vi "Read Multiple Digital Waveforms.vi"(8 "error in (no error)":errorcluster, 9 "Timeout (10000 ms)":u32=10000, 10 "Channels":u16[](array[ring])=[0, 1] items=["POD 1", "POD 2"], 11 "VISA resource name":refnum<visa-resource-name>) -> (0 "error out":errorcluster, 2 "Digital Waveform Graph":digitalwaveform[](graph), 3 "VISA resource name out":refnum<visa-resource-name>)   [LabVIEW 2021, in "Agilent 6000 Series.lvlib"]
doc: "Initiates an acquisition on channel that you enabled with the <B>Configure Digital Channel</B> VI. The VI waits for the acquisition to complete and returns the waveform for the Source channel you specified. If the oscilloscope did not complete the acquisition within the time period you specify with the Timeout parameter, the VI returns a time out error. A common cause for a timeout error is the acquisition was not triggered. For example, the trigger level is out of range of the waveform.\n\nCall the <B>Fetch Digital Waveform</B> VI to obtain the waveforms for each of the remaining enabled Source channels without initiating another acquisition.\n\n<B>NOTE:</B>\n\nThis VI is only supported by MSO models; running this VI with a DSO model might throw an error."
uses:
  Agilent 6000 Series.lvlib
  Low Data VIs/Fetch Digital Waveform.vi
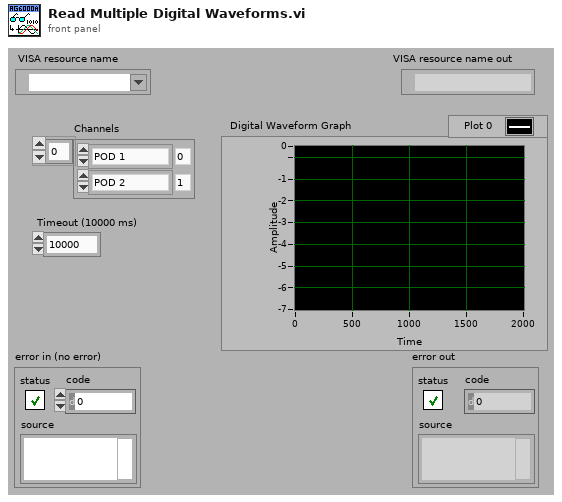
[diagram p1: front panel]
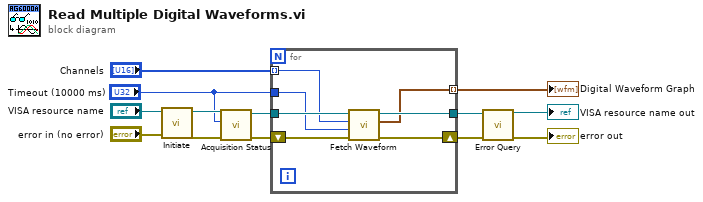
[diagram p0: block diagram]
diagram:
  n1 = call "Initiate.vi"("error in (no error)"="error in (no error)", "VISA resource name"="VISA resource name") -> ("error out"=w6:errorcluster, "VISA resource name out"=w7:refnum<visa-resource-name>)  [unwired: 8 in]
  n2 = call "Acquisition Status.vi"("error in (no error)"=w6, "Timeout (10000 ms)"="Timeout (10000 ms)", "VISA resource name"=w7) -> ("error out"=w5:errorcluster, "VISA resource name out"=w4:refnum<visa-resource-name>)  [unwired: 6 in, 1 out]
  n3 = for {
    tunnel: [w20] -> w9
    tunnel: w4 -> [w17]
    tunnel: "Timeout (10000 ms)" -> [w16]
    tunnel: "Channels" -> [w15] mode=indexing
    tunnel: [w14] -> w1 mode=indexing
    shift-right: [w19] -> w8
    shift-left: w5 -> [w18]
    n4 = call-poly "Fetch Waveform.vi"("error in (no error)"=w18, "Timeout (10000 ms)"=w16, "Source (0: POD 1)"=w15, "VISA resource name"=w17) -> ("error out"=w19:errorcluster, "Digital Waveform Graph"=w14:digitalwaveform, "VISA resource name out"=w20:refnum<visa-resource-name>)  [unwired: 5 in]
  }
  "Digital Waveform Graph" <- w1
  n5 = call "Error Query.vi"("error in (no error)"=w8, "VISA resource name"=w9) -> ("error out"=→"error out":errorcluster, "VISA resource name out"=→"VISA resource name out":refnum<visa-resource-name>)  [unwired: 6 in, 2 out]
